vi "Format SQL INSERT Multivalue.vi"(6 "Times":variant, 8 "error in":errorcluster, 9 "Data":variant, 10 "Path(s)":variant, 11 "Data.PG in":refnum<class "LV-Data.PGSQL.lvclass">) -> (0 "error out":errorcluster, 2 "SQL":string, 3 "Data.PG out":refnum<class "LV-Data.PGSQL.lvclass">, 4 "Paths out":string)   [LabVIEW 2019, in "LV-Data.PGSQL.lvclass"]
uses:
  LV-Data.PGSQL.lvclass
  Typedefs/Errors--enum.ctl
  <vilib>/JDP Science/PostgreSQL Library/Connection/PQ Connection.lvclass
  <vilib>/Utility/Data Type/NI_Data Type.lvlib
  <userlib>/_OpenG.lib/string/string.llb/Trim Whitespace (String)__ogtk.vi
  <vilib>/JDP Science/PostgreSQL Library/Connection/Execute Command (No results).vi
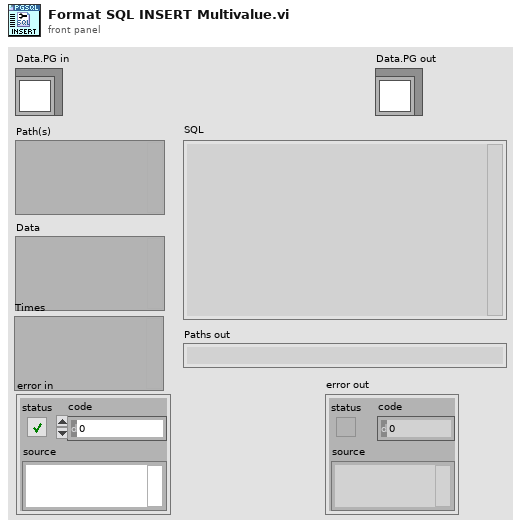
[diagram p1: front panel]
types:
  T1 = typedef "LV-Data.PGSQL.lvclass/Errors--enum.ctl" = enum16{"0: None", "5005: Path Type Not Supported", "5006: Number of Variables", "5007: Number of data points", "5008: Cannot write two data points", "5030: Start and End Times Identical", "5031: Input is not wholly", "5032: Undefined Timestamps", "5033: Bad path or paths", "5040: Invalid Instrument Name", "5050: Column can only hold string", "5051: Column can only hold bool", "5052: Column can only hold double", "5053: Column can only hold int"}
  T2 = typedef "NI_Data Type.lvlib/Data Type.ctl" = enum8{"Invalid Type", "Void", "I8", "I16", "I32", "I64", "U8", "U16", "U32", "U64", "Single Float", "Double Float", "Extended Float", "Single Complex", "Double Complex", "Extended Complex", "Enum U8", "Enum U16", "Enum U32", "Enum U64", "Single Float With Unit", "Double Float With Unit", "Extended Float With Unit", "Single Complex with Unit", "Double Complex with Unit", "Extended Complex with Unit", "Boolean", "String", "Path", "Picture", "Tag", "Array", "Cluster", "Variant", "LV Variant", "Waveform", "Timestamp", "Digital Waveform", "Digital Data", "ExpressData", "Refnum", "External Data", "VI", "Poly VI", "LabVIEW Class Instance", "Fixed Point", "Set Collection", "Map Collection"}
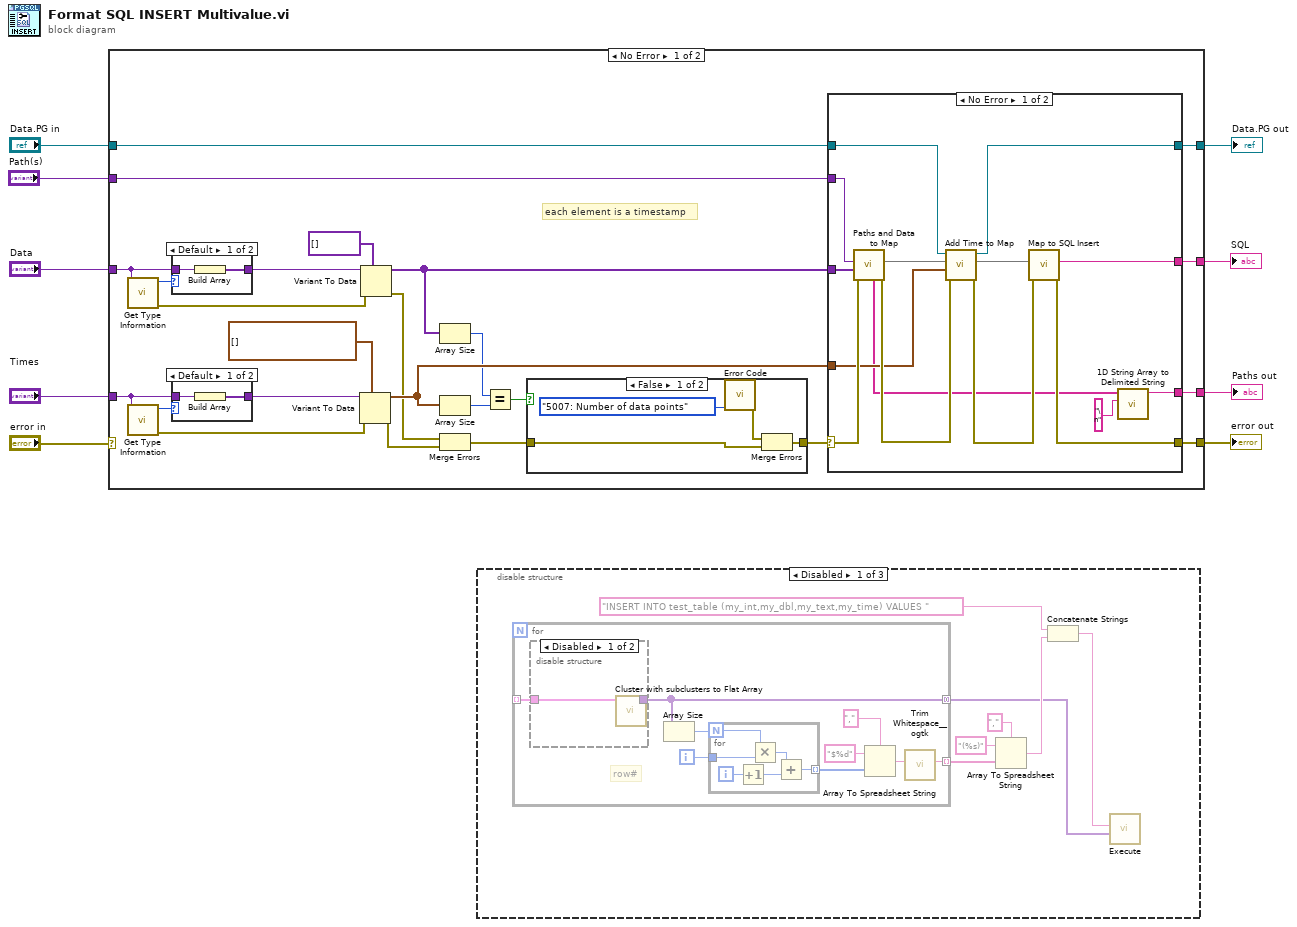
[diagram p0: block diagram]
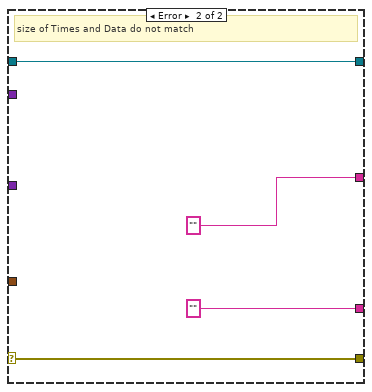
[diagram p5: hidden frame]
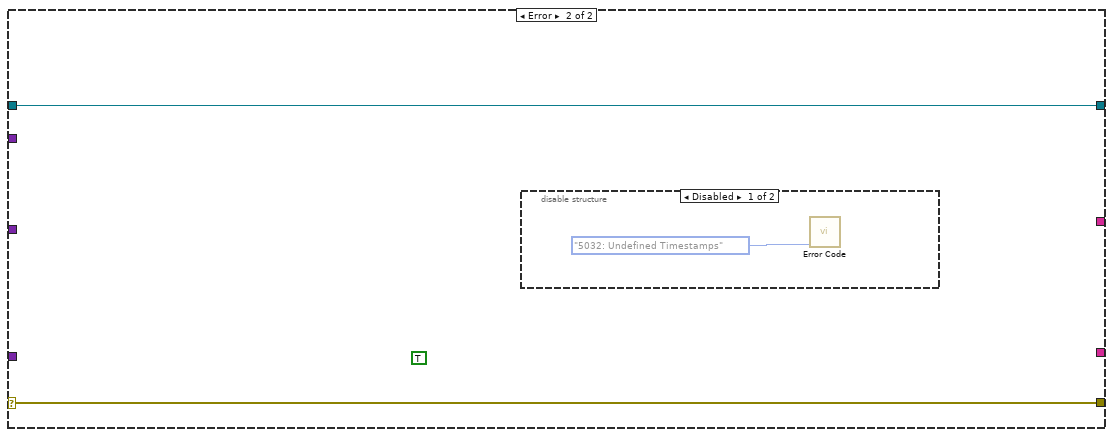
[diagram p6: hidden frame]
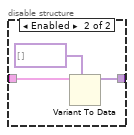
[diagram p8: hidden frame]
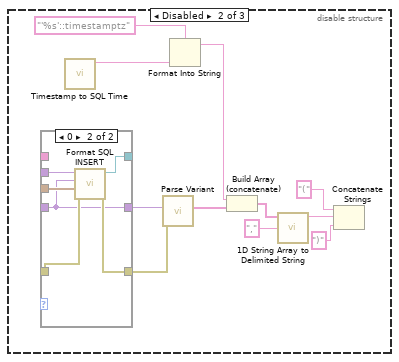
[diagram p9: hidden frame]
diagram:
  n1 = case shown="No Error" "error in" {
    selector: "error in" -> [_ w65]
    tunnel: [w34 w65] -> w9
    tunnel: "Path(s)" -> [w30 _]
    tunnel: [w33 _] -> w8
    tunnel: "Times" -> [w25 _]
    tunnel: [w32 _] -> w1
    tunnel: "Data" -> [w23 _]
    tunnel: "Data.PG in" -> [w29 w66]
    tunnel: [w28 w66] -> w2
    frame No Error {
      # "each element is a timestamp"
      n2 = call <vilib>:"Get Type Information.vi"("variant"=w23) -> ("error out"=w12:errorcluster, "type"=w24:T2)  [unwired: 6 in, 3 out]
      n3 = call <vilib>:"Get Type Information.vi"("variant"=w25) -> ("error out"=w21:errorcluster, "type"=w27:T2)  [unwired: 6 in, 3 out]
      n4 = case shown="Default" w24 {
        tunnel: w23 -> [w41 w42]
        tunnel: [w40 w42] -> w22
        frame Default {
          n5 = Build Array(w41) -> (w40:variant[])
        }
        frame "Array" {
        }
      }
      n6 = case shown="Default" w27 {
        tunnel: w25 -> [w44 w45]
        tunnel: [w43 w45] -> w26
        frame Default {
          n7 = Build Array(w44) -> (w43:variant[])
        }
        frame "Array" {
        }
      }
      n8 = Variant To Data(error in=w21, type=timestamp[] [] ("Times"), Variant=w26) -> (data=w18:timestamp[], error out=w13:errorcluster)
      n9 = Variant To Data(error in=w12, type=variant[] [], Variant=w22) -> (data=w17:variant[], error out=w11:errorcluster)
      n10 = Array Size(array=w17) -> (size(s)=w14:i32)
      n11 = Array Size(array=w18) -> (size(s)=w15:i32)
      n12 = Merge Errors(w11, w13) -> (w10:errorcluster)
      n13 = Equal?(x=w14, y=w15) -> (x = y?=w20:bool)
      n14 = case shown="False" w20 {
        tunnel: [w36 w39] -> w19
        tunnel: w10 -> [w35 w39]
        frame False {
          n15 = call "Error Code.vi"("Error code"=Errors--enum."5007: Number of data points") -> ("error out"=w37:errorcluster)  [unwired: 10 in]
          n16 = Merge Errors(w37, w35) -> (w36:errorcluster)
        }
        frame True {
        }
      }
      n17 = case shown="No Error" w19 {
        selector: w19 -> [w60 w64]
        tunnel: [w51 w64] -> w34
        tunnel: [w50 ""] -> w33
        tunnel: [w46 "" ("delimited string")] -> w32
        tunnel: w30 -> [w57 _]
        tunnel: w18 -> [w56 _]
        tunnel: w17 -> [w59 _]
        tunnel: w29 -> [w49 w61]
        tunnel: [w54 w61] -> w28
        frame No Error {
          n18 = call "Paths and Data to Map.vi"("error in"=w60, "Data"=w59, "Paths"=w57) -> ("error out"=w58:errorcluster, "map out"=w55:map{string, map{string, string[]}}, "paths"=w47:string[])  [unwired: 6 in]
          n19 = call "Add Time to Map.vi"("error in (no error)"=w58, "Times"=w56, "map in"=w55, "LV-Data.PGSQL in"=w49) -> ("error out"=w52:errorcluster, "map out"=w53:map{string, map{string, string[]}}, "LV-Data.PGSQL out"=w54:refnum<class "LV-Data.PGSQL.lvclass">)  [unwired: 5 in]
          n20 = call "Map to SQL Insert.vi"("error in (no error)"=w52, "map in"=w53) -> ("error out"=w51:errorcluster, "delimited string"=w50:string)  [unwired: 8 in]
          n21 = call <vilib>:"1D String Array to Delimited String.vi"("delimiter"="\n", "string array"=w47) -> ("delimited string"=w46:string)  [unwired: 9 in]
        }
        frame Error {
          # "size of Times and Data do not match"
        }
      }
    }
    frame Error {
      (unwired) TRUE
      n22 = disable-structure shown="Disabled" {
        frame Disabled {
          n23 = call "Error Code.vi"("Error code"=Errors--enum."5032: Undefined Timestamps") -> ()  [unwired: 10 in, 1 out]
        }
        frame Enabled {
        }
      }
    }
  }
  "error out" <- w9
  "SQL" <- w8
  "Paths out" <- w1
  "Data.PG out" <- w2
  n24 = disable-structure shown="Disabled" {
    frame Disabled {
      n25 = for {
        tunnel: _ -> [w87] mode=indexing
        tunnel: [w81] -> w76 mode=indexing
        tunnel: [w80] -> w68 mode=concatenating
        i -> [w86]
        # "row#"
        n26 = disable-structure shown="Disabled" {
          disable-tunnel: w87 -> [w89 w92]
          disable-tunnel: [w88 w91] -> w80
          frame Disabled {
            n27 = call <vilib>:"Cluster with subclusters to Flat Array.vi"("Variant"=w89) -> ("Array of items"=w88:variant[])  [unwired: 8 in, 2 out]
          }
          frame Enabled {
            n28 = Variant To Data(type=variant[] [], Variant=w92) -> (data=w91:variant[])  [unwired: 1 in, 1 out]
          }
        }
        n29 = Array Size(array=w80) -> (size(s)=w79:i32)
        n30 = for {
          N: w79 -> [w93]
          tunnel: w86 -> [w97]
          tunnel: [w95] -> w85 mode=indexing
          i -> [w98]
          n31 = Increment(x=w98) -> (x+1=w94:i32)
          n32 = Multiply(x=w93, y=w97) -> (x*y=w96:i32)
          n33 = Add(x=w96, y=w94) -> (x+y=w95:i32)
        }
        n34 = Array To Spreadsheet String(delimiter (Tab)=",", array=w85, 3:"$%d" ("format string")) -> (spreadsheet string=w82:string)
        n35 = call-poly <userlib>:"Trim Whitespace__ogtk.vi"("String in"=w82) -> ("String out"=w81:string)  [unwired: 6 in]
      }
      n36 = Array To Spreadsheet String(delimiter (Tab)=",", array=w76, 3:"(%s)" ("format string")) -> (spreadsheet string=w74:string)
      n37 = Concatenate Strings("INSERT INTO test_table (my_int,my_dbl,my_text,my_time) VALUES " ("command"), w74) -> (w69:string)
      n38 = call-poly <vilib>:"Execute.vi"("Parameters"=w68, "SQL"=w69) -> ("error out"=w71:errorcluster, "PQ Connection out"=w72:refnum<class "PQ Connection.lvclass">, "error in (no error)"=w70:errorcluster, "PQ Connection in"=w73:refnum<class "PQ Connection.lvclass">)  [unwired: 6 in]
    }
    frame Disabled {
      n39 = case shown="0" {
        selector: _ -> [_ _]
        tunnel: _ -> [_ w122]
        tunnel: _ -> [_ w121]
        tunnel: _ -> [w115 w120]
        tunnel: [w114 w119] -> w111
        tunnel: [w115 w118] -> w110
        tunnel: _ -> [w116 w117]
        tunnel: [w116 w117] -> w100
        tunnel: _ -> [w114 _]
        frame Default {
        }
        frame 0 {
          n40 = call "Format SQL INSERT.vi"("error in"=w120, "Data"=w121, "Path(s)"=w117, "LV-Data.PGSQL in"=w122) -> ("error out"=w118:errorcluster, "LV-Data.PGSQL out"=w119:refnum<class "LV-Data.PGSQL.lvclass">)  [unwired: 4 in, 2 out]
        }
      }
      n41 = call "Timestamp to SQL Time.vi"() -> ("date/time string"=w108:string, "Timestamp"=w113:timestamp)  [unwired: 10 in]
      n42 = call "Parse Variant.vi"("error in"=w110, "Data"=w100) -> ("error out"=w99:errorcluster, "Data"=w112:string[])  [unwired: 5 in, 3 out]
      n43 = Format Into String(format string="'%s'::timestamptz" ("delimiter (Tab)"), w108) -> (resulting string=w107:string)  [unwired: 2 in, 1 out]
      n44 = Build Array (concatenate)(w107, w112) -> (w106:string[])
      n45 = call <vilib>:"1D String Array to Delimited String.vi"("delimiter"="," ("delimiter (Tab)"), "string array"=w106) -> ("delimited string"=w104:string)  [unwired: 9 in]
      n46 = Concatenate Strings("(" ("string"), w104, ")" ("string")) -> (w101:string)
    }
    frame Enabled {
    }
  }
